vi "Query Module Serial Number.vi"(8 "error in (no error)":errorcluster, 10 "Platform Slot Number (10)":i16=10 min=-1 max=255, 11 "VISA resource name":refnum<visa-resource-name>) -> (0 "error out":errorcluster, 2 "Serial Number":string, 3 "VISA resource name out":refnum<visa-resource-name>)   [LabVIEW 2018, in "LTB-1.lvlib" / "3150.lvlib"]
doc: "Reads the module's serial number."
uses:
  3150.lvlib
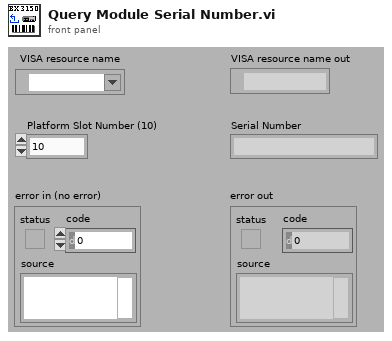
[diagram p1: front panel]
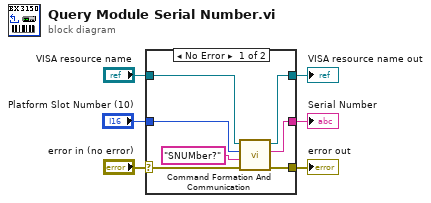
[diagram p0: block diagram]
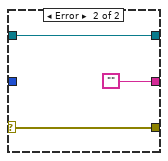
[diagram p2: hidden frame]
diagram:
  n1 = case shown="No Error" "error in (no error)" {
    selector: "error in (no error)" -> [w13 w16]
    tunnel: [w12 w16] -> w1
    tunnel: [w10 w15] -> w5
    tunnel: "VISA resource name" -> [w9 w15]
    tunnel: "Platform Slot Number (10)" -> [w8 _]
    tunnel: [w7 ""] -> w6
    frame No Error {
      n2 = call "Command Formation And Communication.vi"("error in (no error)"=w13, "Command"="SNUMber?", "Platform Slot Number"=w8, "VISA resource name"=w9) -> ("error out"=w12:errorcluster, "Response"=w7:string, "VISA resource name out"=w10:refnum<visa-resource-name>)  [unwired: 5 out]
    }
    frame Error {
    }
  }
  "Serial Number" <- w6
  "VISA resource name out" <- w5
  "error out" <- w1
